vi "Rotation_CreateXY.vi"(9 "Y or sine":dbl, 11 "X or  cosine":dbl) -> (3 "ROTATION":T1)   [LabVIEW 2019, in "PathExecution_Library.lvlib"]
uses:
  PathExecution_Library.lvlib
  ROTATION.ctl
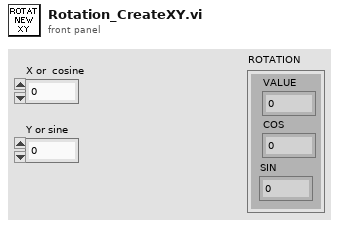
[diagram p1: front panel]
types:
  T1 = typedef "PathExecution_Library.lvlib/ROTATION.ctl" = cluster{"VALUE":dbl, "COS":dbl, "SIN":dbl}
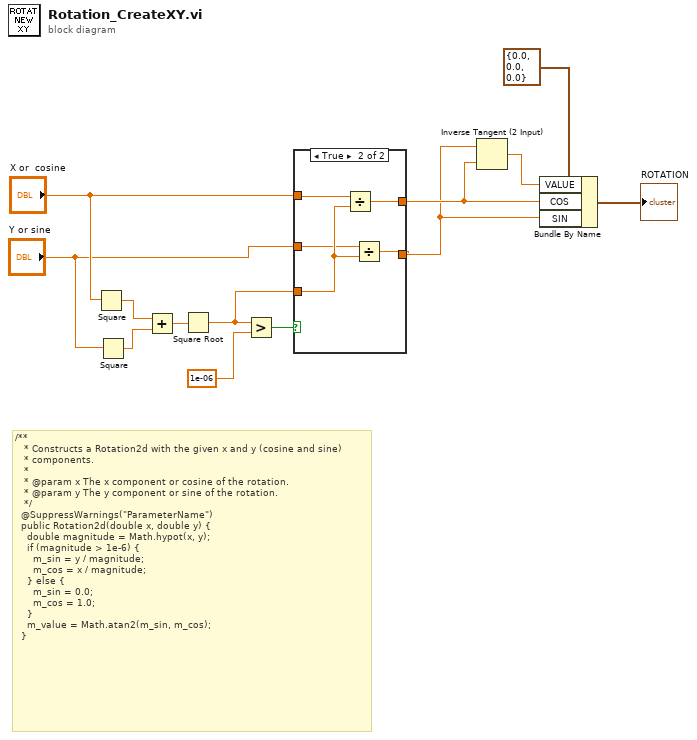
[diagram p0: block diagram]
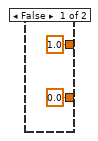
[diagram p2: hidden frame]
diagram:
  # "/**\n   * Constructs a Rotation2d with the given x and y (cosine and sine)\n   * components.\n   *\n   * @param x The x component or cosine of the rotation.\n   * @param y The y component or sine of the rotation.\n   */\n  @SuppressWarnings(\"ParameterName\")\n  public Rotation2d(double x, double y) {\n    double magnitude = Math.hypot(x, y);\n    if (magnitude > 1e-6) {\n      m_sin = y / magnitude;\n      m_cos = x / magnitude;\n    } else {\n      m_sin = 0.0;\n      m_cos = 1.0;\n    }\n    m_value = Math.atan2(m_sin, m_cos);\n  }"
  n1 = Square(x="X or  cosine") -> (x^2=w11:dbl)
  n2 = Square(x="Y or sine") -> (x^2=w10:dbl)
  n3 = Add(x=w11, y=w10) -> (x+y=w9:dbl)
  n4 = Square Root(x=w9) -> (sqrt(x)=w5:dbl)
  n5 = Greater?(x=w5, y=1e-06) -> (0:w7:bool)
  n6 = case shown="True" w7 {
    tunnel: "X or  cosine" -> [_ w20]
    tunnel: w5 -> [_ w19]
    tunnel: [1.0 w18] -> w3
    tunnel: "Y or sine" -> [_ w17]
    tunnel: [0.0 w16] -> w2
    frame False {
    }
    frame True {
      n7 = Divide(x=w20, y=w19) -> (x/y=w18:dbl)
      n8 = Divide(x=w17, y=w19) -> (x/y=w16:dbl)
    }
  }
  n9 = Inverse Tangent (2 Input)(1:w3, 2:w2) -> (0:w1:dbl)
  n10 = Bundle By Name(cluster=T1 {"VALUE"=0.0, "COS"=0.0, "SIN"=0.0} ("ROTATION"), "VALUE"=w1, "COS"=w3, "SIN"=w2) -> (→"ROTATION":T1)
